vi "XY Graph Compare X Array.vi"(2 "Plot Array":cluster{"Array":dbl[], "Array":dbl[]}[](array[cluster])) -> (7 "Same [X]?":bool)   [LabVIEW 2019]
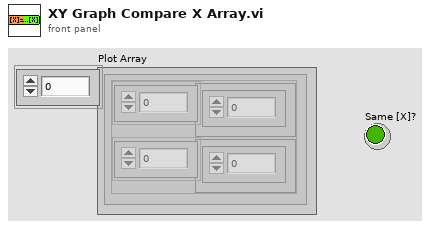
[diagram p1: front panel]
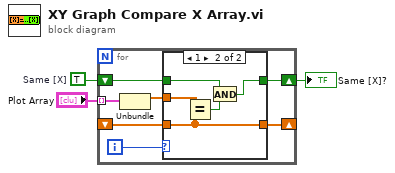
[diagram p0: block diagram]
diagram:
  w2 = TRUE  # Same [X]
  n1 = for {
    tunnel: "Plot Array" -> [w10] mode=indexing
    shift-right: [w7] -> _
    shift-left: _ -> [w6]
    shift-right: [w4] -> w1
    shift-left: w2 -> [w5]
    i -> [w9]
    n2 = Unbundle(w10) -> ("Array"=w8:dbl[])  [unwired: 1 out]
    n3 = case shown="1" w9 {
      tunnel: w8 -> [w12 w17]
      tunnel: [w12 w16] -> w7
      tunnel: w6 -> [_ w16]
      tunnel: w5 -> [w11 w15]
      tunnel: [w11 w13] -> w4
      frame 0, Default {
      }
      frame 1 {
        n4 = Equal?(x=w17, y=w16) -> (x = y?=w14:bool)
        n5 = And(x=w15, y=w14) -> (x .and. y?=w13:bool)
      }
    }
  }
  "Same [X]?" <- w1
